vi "createGObject.vi"(8 "error in (no error)":errorcluster, 10 "GObjectSelection":T1, 11 "IGObjectFactory in":refnum<class "IGObjectFactory.lvclass">) -> (0 "error out":errorcluster, 2 "GObject":refnum<class "GObject.lvclass">, 3 "IGObjectFactory out":refnum<class "IGObjectFactory.lvclass">)   [LabVIEW 2016, in "IGObjectFactory.lvclass"]
uses:
  IGObjectFactory.lvclass
  Typedefs/GObjectSelection.ctl
  GObject/GObject.lvclass
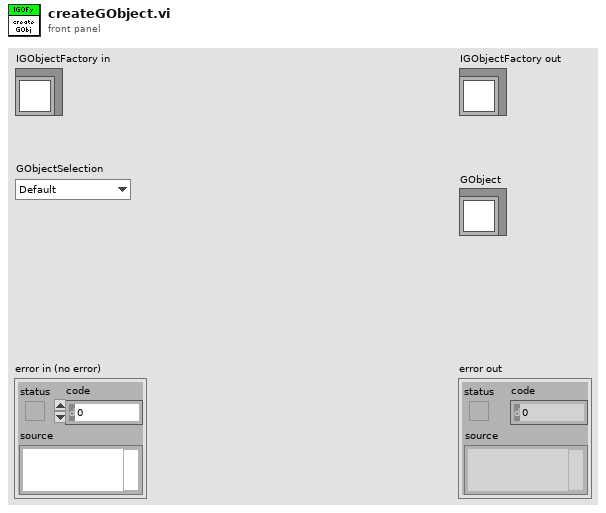
[diagram p1: front panel]
types:
  T1 = typedef "GObjectSelection.ctl" = enum16{"Default", "CaseStructure", "ClusterConstant", "EnumConstant", "EventStructure", "FlatSequence", "ForLoop", "WhileLoop"}
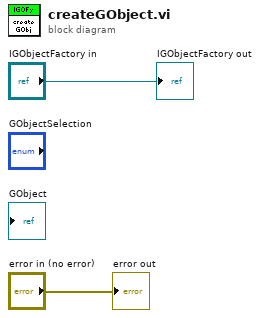
[diagram p0: block diagram]
diagram:
  "error out" <- "error in (no error)"
  "IGObjectFactory out" <- "IGObjectFactory in"
